vi "ADC Read.vi"() -> (3 "Data out":T1[](array[typedef]))   [LabVIEW 2025]
uses:
  <instrlib>/_niInstr/DSP/v1/Shared/Public/IQ Data.ctl
  <vilib>/rvi/eio/common/nirviEmuTemplateMethod_errors.vi
  <instrlib>/_niInstr/DSP/v1/FPGA/Public/Sub VIs/Data Conversion/I16 to IQ - 1 spc - S18.1.vi
  <vilib>/eio/EIONode/EIONode.xnode
  <instrlib>/_niInstr/DSP/v1/FPGA/niInstr DSP v1 FPGA.lvlib
  <instrlib>/_niInstr/DSP/v1/Shared/niInstr DSP v1 Shared.lvlib
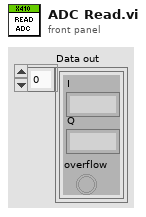
[diagram p1: front panel]
types:
  T1 = typedef "niInstr DSP v1 Shared.lvlib/IQ Data.ctl" = cluster{"I":fxp<+/-,18,1>, "Q":fxp<+/-,18,1>, "overflow":bool}
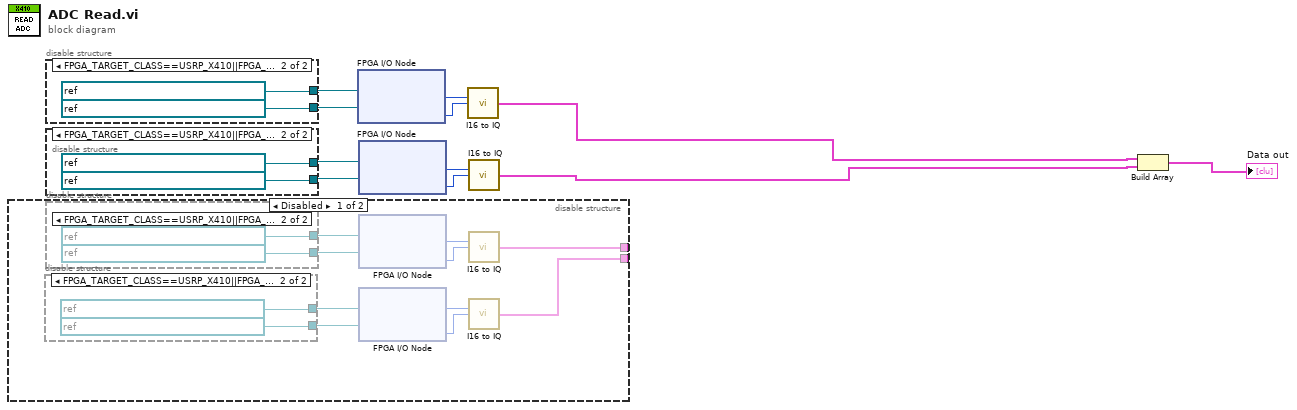
[diagram p0: block diagram]
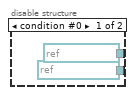
[diagram p2: hidden frame]
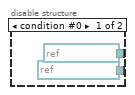
[diagram p3: hidden frame]
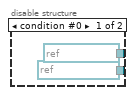
[diagram p5: hidden frame]
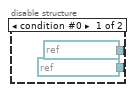
[diagram p6: hidden frame]
diagram:
  n1 = disable-structure shown="Disabled" {
    disable-tunnel: [w13 _] -> _
    disable-tunnel: [w12 _] -> _
    frame Disabled {
      n2 = disable-structure shown="FPGA_TARGET_CLASS==USRP_X410||FPGA_TARGET_CLASS==USRP_X410__EMBEDDED____UNSUPPORTED" {
        disable-tunnel: [refnum<k21> "RF 0/Rx/Q" ("FPGA I/O In") refnum<k21> "Daughterboard 1\\RF 1.Rx.Q" ("FPGA I/O In")] -> w17
        disable-tunnel: [refnum<k21> "RF 0/Rx/I" ("FPGA I/O In") refnum<k21> "Daughterboard 1\\RF 1.Rx.I" ("FPGA I/O In")] -> w16
        frame condition #0 {
        }
        frame condition #1 (active) {
        }
      }
      n3 = disable-structure shown="FPGA_TARGET_CLASS==USRP_X410||FPGA_TARGET_CLASS==USRP_X410__EMBEDDED____UNSUPPORTED" {
        disable-tunnel: [refnum<k21> "RF 0/Rx/Q" ("FPGA I/O In") refnum<k21> "Daughterboard 1\\RF 0.Rx.Q" ("FPGA I/O In")] -> w15
        disable-tunnel: [refnum<k21> "RF 0/Rx/I" ("FPGA I/O In") refnum<k21> "Daughterboard 1\\RF 0.Rx.I" ("FPGA I/O In")] -> w14
        frame condition #0 {
        }
        frame condition #1 (active) {
        }
      }
      n4 = xnode "FPGA I/O Node"("FPGA I/O In"=w14, "FPGA I/O In"=w15) -> ("I/O Item"=w21:i16, "I/O Item"=w20:i16)  [unwired: 2 out]
      n5 = xnode "FPGA I/O Node"("FPGA I/O In"=w16, "FPGA I/O In"=w17) -> ("I/O Item"=w19:i16, "I/O Item"=w18:i16)  [unwired: 2 out]
      n6 = call-poly <instrlib>:"I16 to IQ.vi"("I"=w21, "Q"=w20) -> ("IQ"=w13:T1)  [unwired: 13 in]
      n7 = call-poly <instrlib>:"I16 to IQ.vi"("I"=w19, "Q"=w18) -> ("IQ"=w12:T1)  [unwired: 13 in]
    }
    frame Enabled {
    }
  }
  n8 = disable-structure shown="FPGA_TARGET_CLASS==USRP_X410||FPGA_TARGET_CLASS==USRP_X410__EMBEDDED____UNSUPPORTED" {
    disable-tunnel: [refnum<k21> "RF 0/Rx/Q" ("FPGA I/O In") refnum<k21> "Daughterboard 0\\RF 0.Rx.Q" ("FPGA I/O In")] -> w3
    disable-tunnel: [refnum<k21> "RF 0/Rx/I" ("FPGA I/O In") refnum<k21> "Daughterboard 0\\RF 0.Rx.I" ("FPGA I/O In")] -> w2
    frame condition #0 {
    }
    frame condition #1 (active) {
    }
  }
  n9 = disable-structure shown="FPGA_TARGET_CLASS==USRP_X410||FPGA_TARGET_CLASS==USRP_X410__EMBEDDED____UNSUPPORTED" {
    disable-tunnel: [refnum<k21> "RF 0/Rx/Q" ("FPGA I/O In") refnum<k21> "Daughterboard 0\\RF 1.Rx.Q" ("FPGA I/O In")] -> w5
    disable-tunnel: [refnum<k21> "RF 0/Rx/I" ("FPGA I/O In") refnum<k21> "Daughterboard 0\\RF 1.Rx.I" ("FPGA I/O In")] -> w4
    frame condition #0 {
    }
    frame condition #1 (active) {
    }
  }
  n10 = xnode "FPGA I/O Node"("FPGA I/O In"=w2, "FPGA I/O In"=w3) -> ("I/O Item"=w9:i16, "I/O Item"=w8:i16)  [unwired: 2 out]
  n11 = xnode "FPGA I/O Node"("FPGA I/O In"=w4, "FPGA I/O In"=w5) -> ("I/O Item"=w7:i16, "I/O Item"=w6:i16)  [unwired: 2 out]
  n12 = call-poly <instrlib>:"I16 to IQ.vi"("I"=w9, "Q"=w8) -> ("IQ"=w10:T1)  [unwired: 13 in]
  n13 = call-poly <instrlib>:"I16 to IQ.vi"("I"=w7, "Q"=w6) -> ("IQ"=w1:T1)  [unwired: 13 in]
  n14 = Build Array(w10, w1) -> (→"Data out":T1[])
